vi "HandlingError.vi"(1 "error input":errorcluster, 2 "reminder":string) -> (0 "error output":errorcluster)   [LabVIEW 2023]
uses:
  GlobalVariant.vi
panel:
  out "appended path":path
  out "date/time string":string
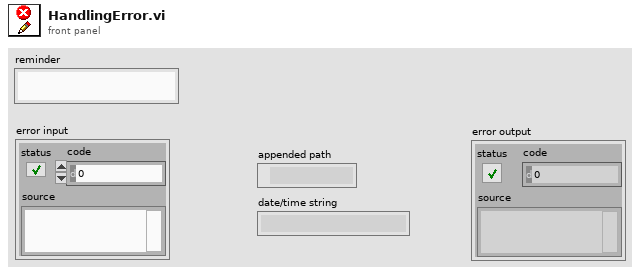
[diagram p1: front panel]
types:
  T1 = enum16{"open", "replace", "create", "open or create", "replace or create", "replace or create with confirmation"}
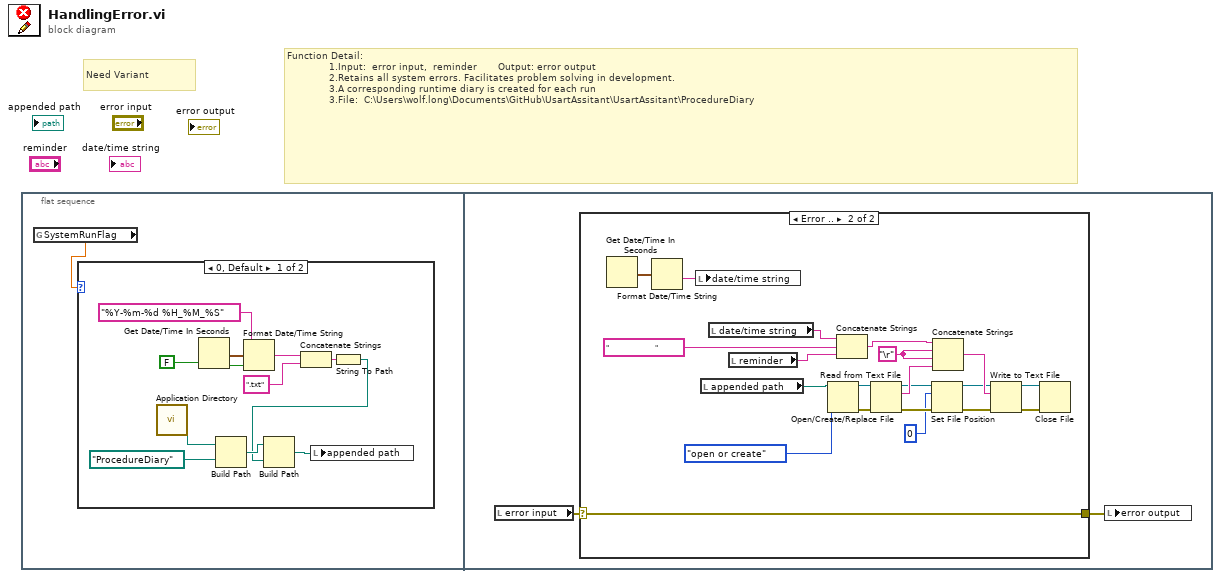
[diagram p0: block diagram]
diagram:
  # "Function Detail:\n              1.Input:  error input,  reminder       Output: error output\n              2.Retains all system errors. Facilitates problem solving in development.\n              3.A corresponding runtime diary is created for each run\n              3.File:  C:\\Users\\wolf.long\\Documents\\GitHub\\UsartAssitant\\UsartAssitant\\ProcedureDiary"
  # "Need Variant"
  n1 = flat-sequence {
    frame #0 {
      n2 = global read "GlobalVariant.vi" "SystemRunFlag"() -> (w1:dbl)
      n3 = case shown="0, Default" w1 {
        frame 0, Default {
          n4 = call <vilib>:"Application Directory.vi"() -> ("Application Directory"=w12:path)
          n5 = Get Date/Time In Seconds() -> (seconds since 1Jan1904=w9:timestamp)
          n6 = Build Path(base path=w12, name or relative path=path "ProcedureDiary") -> (appended path=w11:path)
          n7 = Format Date/Time String(time format string (%c)="%Y-%m-%d %H_%M_%S", seconds (now)=w9, UTC format=FALSE) -> (date/time string=w5:string)
          n8 = Concatenate Strings(w5, ".txt" ("string")) -> (w6:string)
          n9 = String To Path(string=w6) -> (path=w2:path)
          n10 = Build Path(base path=w11, name or relative path=w2) -> (appended path=w7:path)
          n11 = local write "appended path"(w7) -> ()
        }
        frame 1 {
        }
      }
    }
    frame #1 {
      n12 = local read "error input"() -> (w14:errorcluster)
      n13 = case shown="Error .." w14 {
        selector: w14 -> [w15 w19]
        tunnel: [w15 w19] -> w13
        frame No Error {
        }
        frame Error {
          w21 = "\r"
          n14 = Get Date/Time In Seconds() -> (seconds since 1Jan1904=w18:timestamp)
          n15 = Format Date/Time String(seconds (now)=w18) -> (date/time string=w17:string)  [unwired: 2 in]
          n16 = local write "date/time string"(w17) -> ()
          n17 = local read "appended path"() -> (w16:path)
          n18 = local read "date/time string"() -> (w29:string)
          n19 = local read "reminder"() -> (w30:string)
          n20 = Open/Create/Replace File(file path (use dialog)=w16, operation (0:open)=T1."open or create") -> (refnum out=w24:refnum<file>, error out=w33:errorcluster)  [unwired: 4 in, 1 out]
          n21 = Concatenate Strings(w29, "                       " ("string"), w30) -> (w28:string)
          n22 = Read from Text File(file (use dialog)=w24, error in=w33) -> (refnum out=w25:refnum<file>, text=w27:string, error out=w31:errorcluster)  [unwired: 2 in, 1 out]
          n23 = Set File Position(offset (in bytes) (0)=i64 0, refnum=w25, error in=w31) -> (refnum out=w26:refnum<file>, error out=w32:errorcluster)  [unwired: 1 in]
          n24 = Concatenate Strings(w28, w21, w21, w27) -> (w36:string)
          n25 = Write to Text File(file (use dialog)=w26, text=w36, error in=w32) -> (refnum out=w35:refnum<file>, error out=w34:errorcluster)  [unwired: 1 in, 1 out]
          n26 = Close File(refnum=w35, error in=w34) -> ()  [unwired: 2 out]
        }
      }
      n27 = local write "error output"(w13) -> ()
    }
  }
